vi "Command Engine.vi"(10 "Parameters":variant, 11 "Process":refnum<class "Process.lvclass">) -> ()   [LabVIEW 2015, in "J1939 Addon Engine.lvlib"]
uses:
  J1939 Addon Engine.lvlib
  <vilib>/NI/NIVS Inline Async API/_VS Inline Async API/Process/Process.lvclass
  Types/Diagnostic Data Lookup Table Action.ctl
  <vilib>/NI/NIVS Inline Async API/_VS Inline Async API/Process/Process.lvclass/Process.ctl
  Shared/Types/SysDef Command Settings.ctl
  <vilib>/NI/NIVS Inline Async API/_Data Access Engine/Access Type Classes/Read/Read.lvclass/Read.ctl
  <vilib>/NI/NIVS Inline Async API/_Data Access Engine/Access Type Classes/Write/Write.lvclass/Write.ctl
  APIs/Host Automation API/Types/DTC_Action.ctl
  <vilib>/NI/NIVS Inline Async API/_Data Access Engine/Data Access Engine/Methods/Write.Data.vi
  <vilib>/NI/NIVS Inline Async API/_Data Access Engine/Data Access Engine/Methods/Read.Data.vi
  <vilib>/NI/NIVS Inline Async API/_VS Inline Async API/Process/Data Member Access/Read Data Access.vi
  <vilib>/NI/NIVS Inline Async API/_VS Inline Async API/Error Handling Process/SubVIs/Error.ConvertArray.vi
  <vilib>/NI/NIVS Inline Async API/_Data Access Engine/Access Type Classes/Write/Write.ProcessData.vi
  <vilib>/NI/NIVS Inline Async API/_Data Access Engine/Access Type Classes/Read/Read.ProcessData.vi
  Diagnostic Data Lookup Table.vi
  Shared/SubVIs/Constants.vi
  <vilib>/NI/NIVS Inline Async API/_Data Access Engine/Data Access Engine/Methods/Read.Lookup.vi
  <vilib>/NI/NIVS Inline Async API/_Data Access Engine/Data Access Engine/Methods/Write.Lookup.vi
  <vilib>/NI/NIVS Inline Async API/_Data Access Engine/Data Access Engine/Data Access Engine.lvclass
  APIs/Host Automation API/J1939 Host Automation API.lvlib
  Shared/J1939 Addon Shared.lvlib
  <vilib>/NI Veristand/Custom Device Tools/Custom Device Utility Library/Custom Device Utility Library.lvlib
panel:
  in  "Error":errorcluster
  out "error out":errorcluster
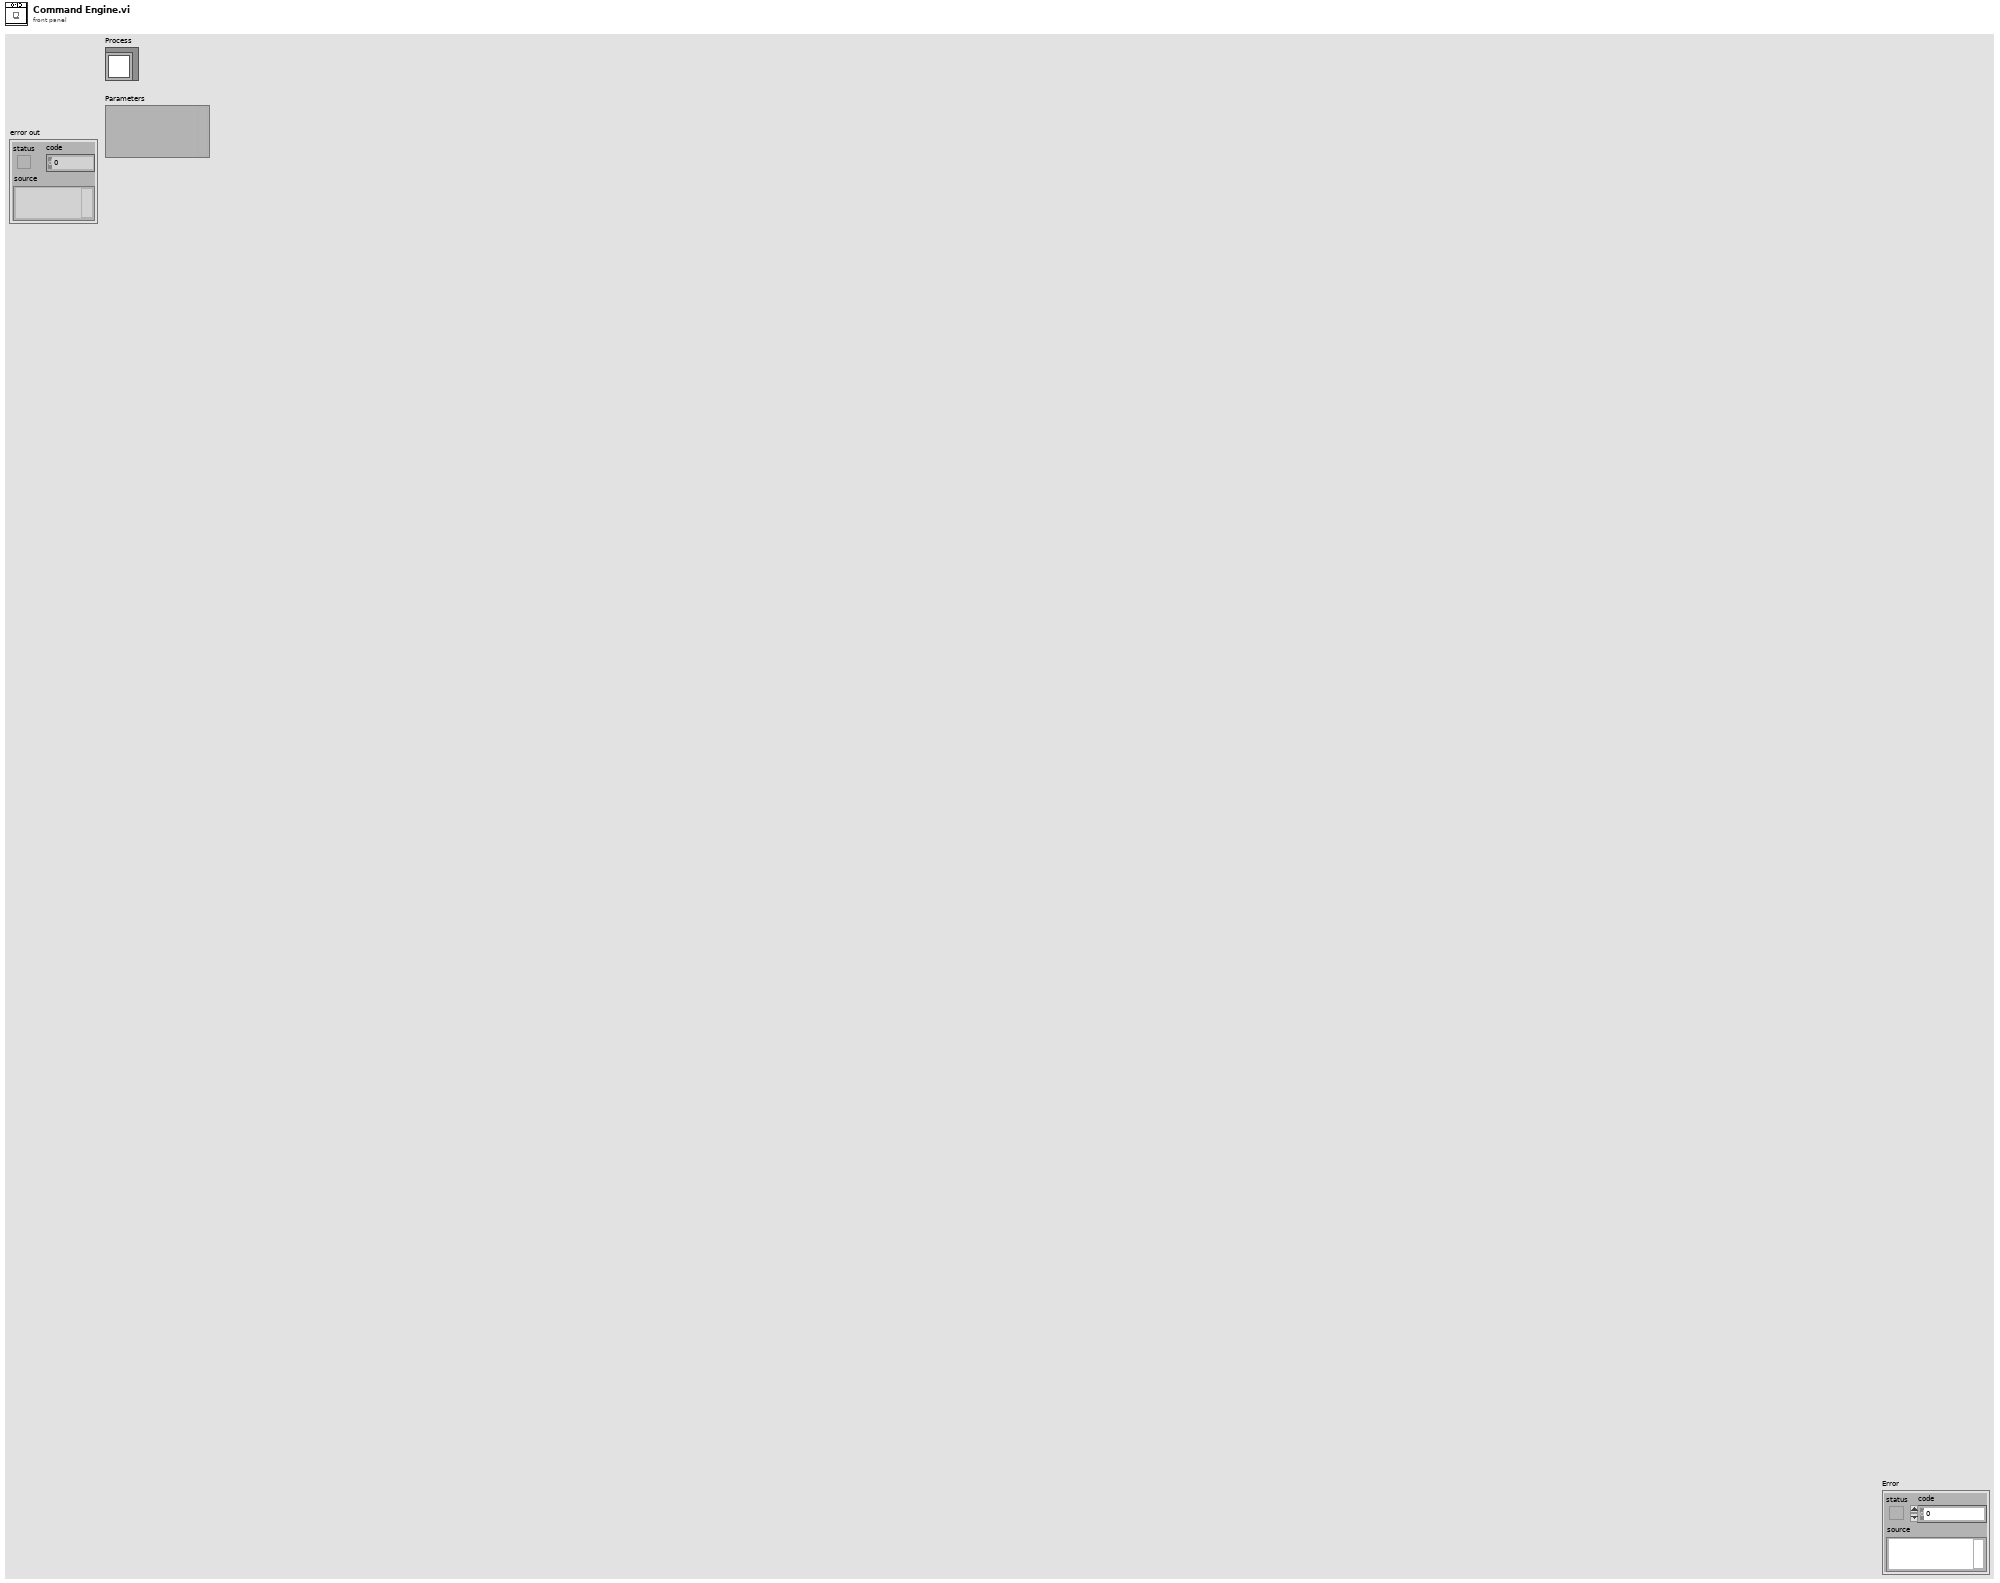
[diagram p1: front panel]
types:
  T1 = typedef "J1939 Addon Shared.lvlib/SysDef Command Settings.ctl" = cluster{"Name":string, "Response Refs":cluster{"Values Array":dbl[], "Response Names":string[]}, "Command Refs":cluster{"Values Array":dbl[], "Command Names":string[]}}
  T2 = typedef "Data Access Engine.lvlib/Data Access Engine.lvclass/Write.DVR.ctl" = refnum<data-value>
  T3 = typedef "Data Access Engine.lvlib/Data Access Engine.lvclass/Read.DVR.ctl" = refnum<data-value>
  T4 = typedef "J1939 Addon Engine.lvlib/Diagnostic Data Lookup Table Reference.ctl" = refnum<data-value>
  T5 = typedef "NI STM.lvlib/TCP Connection Info.ctl" = cluster{"connection ID":refnum<k5>, "meta data":T6[]}
  T6 = typedef "NI STM.lvlib/MetaDataElement.ctl" = string
  T7 = typedef "J1939 Addon Engine.lvlib/Diagnostic Data Lookup Table Action.ctl" = enum16{"Initialize", "Get All", "Set All", "Set Value", "Get Value"}
  T8 = typedef "J1939 Host Automation API.lvlib/DTC_Action.ctl" = enum16{"ALL", "ACTIVE", "INACTIVE"}
  T9 = typedef "J1939 Addon Engine.lvlib/Internal Command Engine States.ctl" = enum8{"Idle", "Refresh Address", "Verify DTCs", "Clear DTCs", "Clear Status Bit", "Clear Error Bit"}
  T10 = typedef "J1939 Host Automation API.lvlib/Verify DTC_Status.ctl" = enum16{"NOT_PRESENT", "ACTIVE", "INACTIVE"}
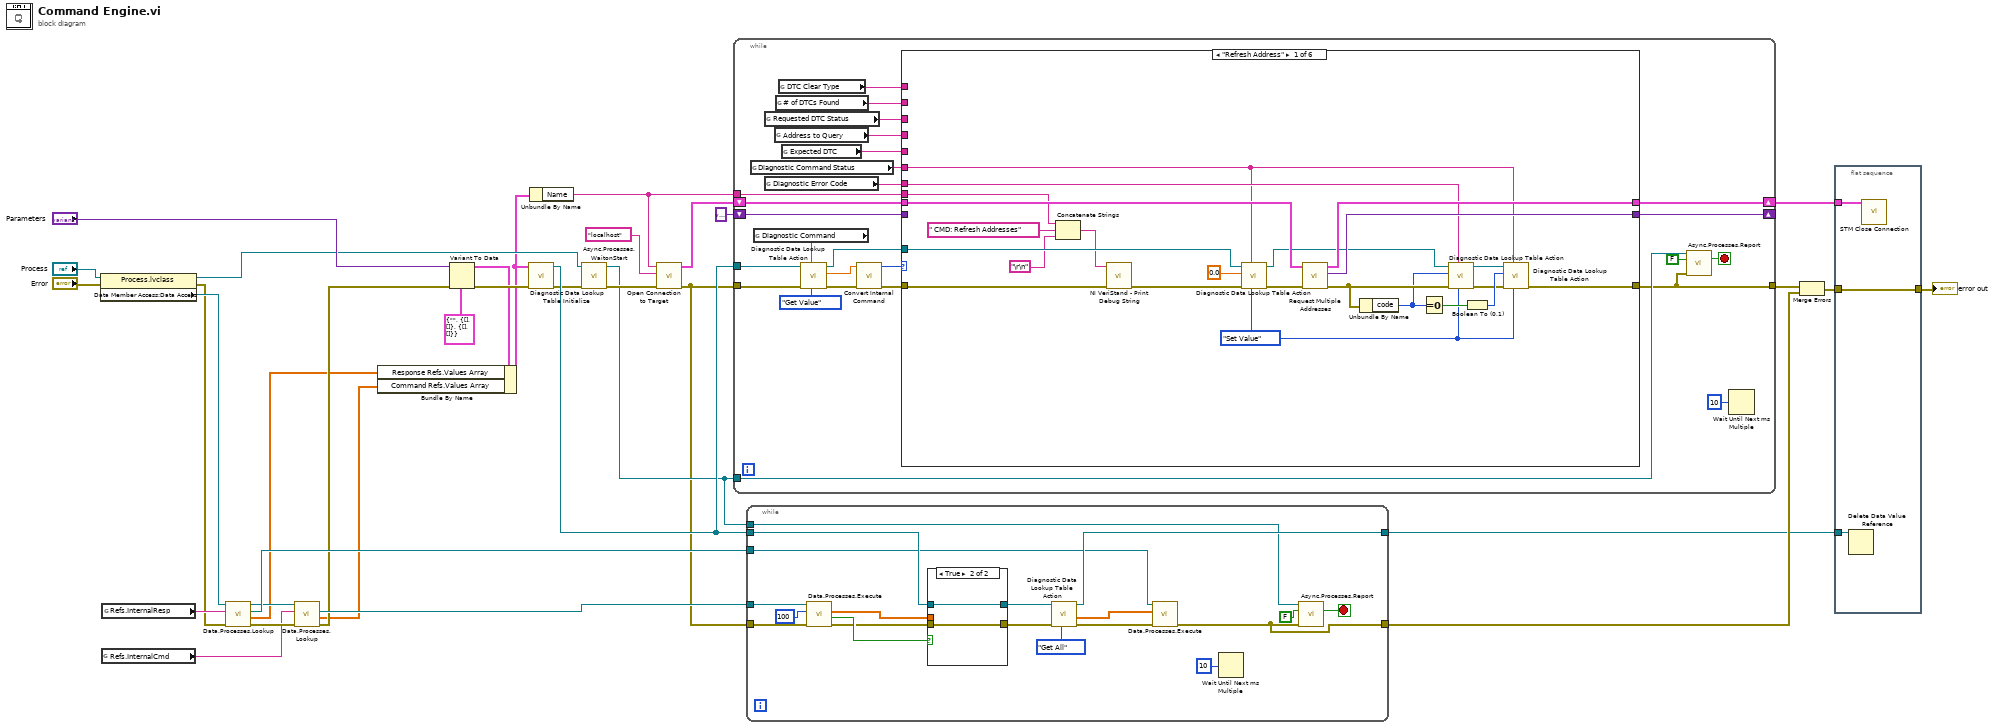
[diagram p0: block diagram]
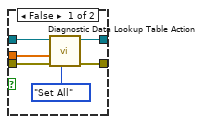
[diagram p2: hidden frame]
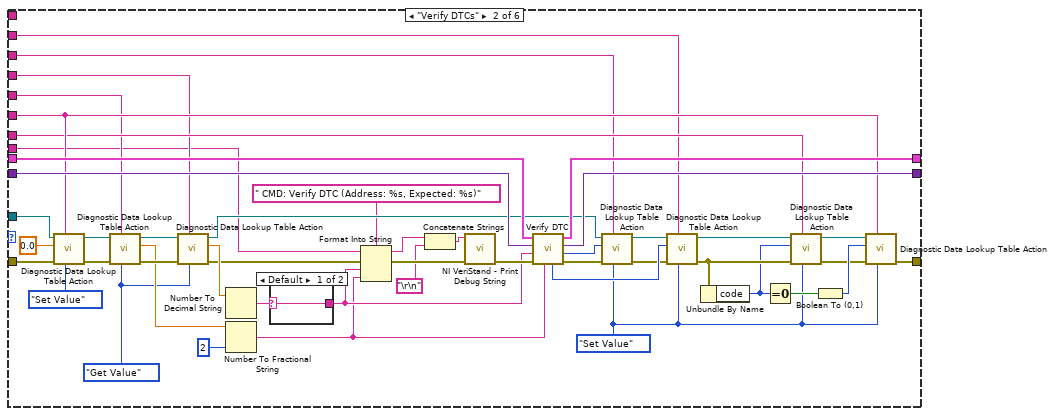
[diagram p3: hidden frame]
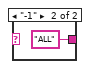
[diagram p4: hidden frame]
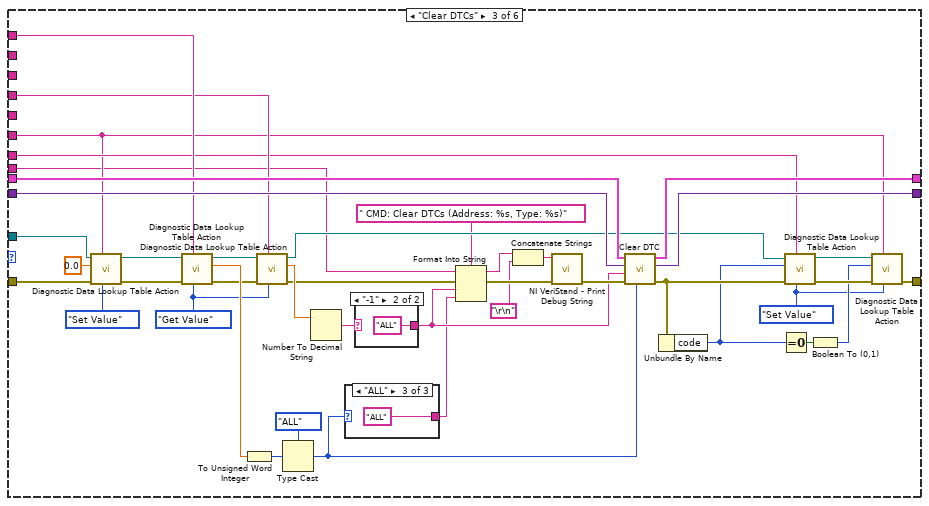
[diagram p5: hidden frame]
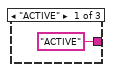
[diagram p6: hidden frame]
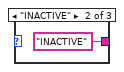
[diagram p7: hidden frame]
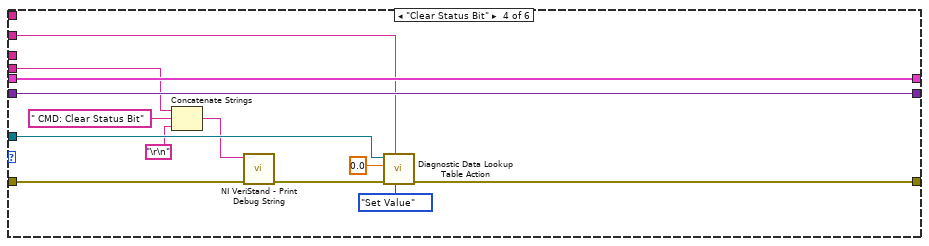
[diagram p9: hidden frame]
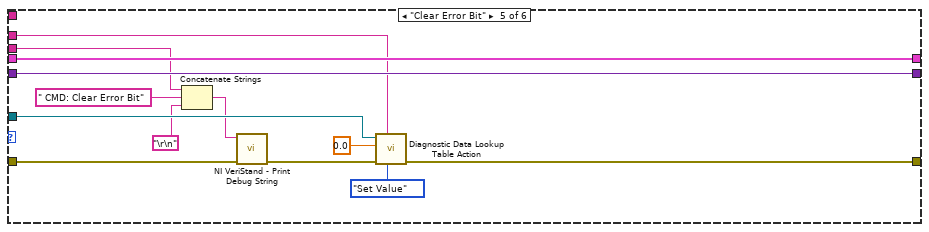
[diagram p10: hidden frame]
diagram:
  n1 = property class="Process.lvclass"(reference="Process", error in="Error") -> (reference out=w18:refnum<class "Process.lvclass">, error out=w10:errorcluster, "Data Member Access:Data Access"=w15:refnum<class "Data Access Engine.lvclass">)
  n2 = global read "Constants.vi" "Refs.InternalCmd"() -> (w13:string)
  n3 = global read "Constants.vi" "Refs.InternalResp"() -> (w12:string)
  n4 = call-poly <vilib>:"Data.Processes.Lookup.vi"("error in (no error)"=w10, "Name"=w12, "Data Access API in"=w15) -> ("error out"=w17:errorcluster, "Initial Values"=w4:dbl[], "Ref"=w20:T2, "Data Access API out"=w16:refnum<class "Data Access Engine.lvclass">)  [unwired: 5 in]
  n5 = call-poly <vilib>:"Data.Processes.Lookup.vi"("error in (no error)"=w17, "Name"=w13, "Data Access API in"=w16) -> ("error out"=w7:errorcluster, "Initial Values"=w3:dbl[], "Ref"=w21:T3)  [unwired: 5 in, 1 out]
  n6 = Variant To Data(error in=w7, type=T1 {"Name"="", "Response Refs"={"Values Array"=[], "Response Names"=[]}, "Command Refs"={"Values Array"=[], "Command Names"=[]}} ("Internal Command Engine References"), Variant="Parameters") -> (data=w5:T1, error out=w8:errorcluster)
  n7 = Bundle By Name(cluster=w5, "Response Refs.Values Array"=w4, "Command Refs.Values Array"=w3) -> (w2:T1)
  n8 = call "Diagnostic Data Lookup Table Initialize.vi"("error in (no error)"=w8, "Internal Command Engine References"=w2) -> ("error out"=w9:errorcluster, "Diag Data Ref"=w31:T4)  [unwired: 8 in]
  n9 = Unbundle By Name(w2) -> ("Name"=w1:string)
  n10 = call <vilib>:"Async.Processes.WaitonStart.vi"("error in (no error)"=w9, "Process"=w18) -> ("error out"=w24:errorcluster, "Process out"=w23:refnum<class "Process.lvclass">)  [unwired: 7 in, 1 out]
  n11 = call "Open Connection to Target.vi"("error in (no error)"=w24, "IP Address"="localhost", "TCP Service"=w1) -> ("error out"=w14:errorcluster, "connection info"=w33:T5)  [unwired: 7 in]
  n12 = while {
    shift-right: [w59] -> _
    shift-left: variant ("Address Lookup Table Out") -> [w58]
    shift-right: [w57] -> w25
    shift-left: w33 -> [w60]
    tunnel: [w35] -> w30
    tunnel: w14 -> [w54]
    tunnel: w23 -> [w52]
    tunnel: w31 -> [w53]
    tunnel: w1 -> [w51]
    stop <- w55 stop-if-true
    n13 = global read "Constants.vi" "Diagnostic Command Status"() -> (w43:string)
    n14 = global read "Constants.vi" "Diagnostic Command"() -> (w45:string)
    n15 = global read "Constants.vi" "Requested DTC Status"() -> (w37:string)
    n16 = global read "Constants.vi" "Diagnostic Error Code"() -> (w41:string)
    n17 = global read "Constants.vi" "Address to Query"() -> (w38:string)
    n18 = global read "Constants.vi" "# of DTCs Found"() -> (w36:string)
    n19 = global read "Constants.vi" "DTC Clear Type"() -> (w40:string)
    n20 = global read "Constants.vi" "Expected DTC"() -> (w39:string)
    n21 = call "Diagnostic Data Lookup Table Action.vi"("command"=Diagnostic_Data_Lookup_Table_Action."Get Value", "Name"=w45, "error in (no error)"=w54, "Diag Data Ref"=w53) -> ("error out"=w47:errorcluster, "Signal Out"=w48:dbl, "Diag Data Ref Out"=w42:T4)  [unwired: 4 in, 1 out]
    n22 = call "Convert Internal Command.vi"("error in (no error)"=w47, "Value"=w48) -> ("error out"=w46:errorcluster, "Enum"=w49:T9)  [unwired: 8 in]
    n23 = case shown="\"Refresh Address\"" w49 {
      tunnel: w60 -> [w83 w131 w175 w192 w205 w208]
      tunnel: [w82 w129 w173 w191 w204 w207] -> w59
      tunnel: w58 -> [_ w130 w174 w191 w204 w207]
      tunnel: [w81 w128 w172 w192 w205 w208] -> w57
      tunnel: w46 -> [w66 w116 w161 w186 w199 w209]
      tunnel: [w76 w112 w163 w190 w203 w209] -> w35
      tunnel: w43 -> [w69 w103 w149 w189 _ _]
      tunnel: w42 -> [w73 w110 w157 w187 w201 _]
      tunnel: w41 -> [w70 w102 w150 _ w202 _]
      tunnel: w40 -> [_ _ w152 _ _ _]
      tunnel: w39 -> [_ w101 _ _ _ _]
      tunnel: w38 -> [_ w100 w151 _ _ _]
      tunnel: w37 -> [_ w99 _ _ _ _]
      tunnel: w36 -> [_ w98 _ _ _ _]
      tunnel: w51 -> [w63 w86 w137 w184 w197 _]
      frame "Refresh Address" {
        w68 = Diagnostic_Data_Lookup_Table_Action."Set Value" ("command")
        n24 = Concatenate Strings(w63, " CMD: Refresh Addresses" ("string"), "\r\n") -> (w62:string)
        n25 = call <vilib>:"NI VeriStand - Print Debug String.vi"("error in (no error)"=w66, "Message"=w62) -> ("error out"=w65:errorcluster)  [unwired: 9 in]
        n26 = call "Diagnostic Data Lookup Table Action.vi"("command"=w68, "Name"=w69, "error in (no error)"=w65, "Signal In"=0.0 ("Value"), "Diag Data Ref"=w73) -> ("error out"=w75:errorcluster, "Diag Data Ref Out"=w72:T4)  [unwired: 3 in, 2 out]
        n27 = call "Request Multiple Addresses.vi"("error in (no error)"=w75, "connection info"=w83) -> ("error out"=w78:errorcluster, "variant"=w82:variant, "connection info"=w81:T5)  [unwired: 6 in, 1 out]
        n28 = Unbundle By Name(w78) -> ("code"=w67:i32)
        n29 = Equal To 0?(x=w67) -> (x = 0?=w80:bool)
        n30 = call "Diagnostic Data Lookup Table Action.vi"("command"=w68, "Name"=w70, "error in (no error)"=w78, "Signal In"=w67, "Diag Data Ref"=w72) -> ("error out"=w77:errorcluster, "Diag Data Ref Out"=w71:T4)  [unwired: 3 in, 2 out]
        n31 = Boolean To (0,1)(Boolean=w80) -> (0, 1=w79:i16)
        n32 = call "Diagnostic Data Lookup Table Action.vi"("command"=w68, "Name"=w69, "error in (no error)"=w77, "Signal In"=w79, "Diag Data Ref"=w71) -> ("error out"=w76:errorcluster)  [unwired: 3 in, 3 out]
      }
      frame "Verify DTCs" {
        w95 = Diagnostic_Data_Lookup_Table_Action."Set Value" ("command")
        w97 = Diagnostic_Data_Lookup_Table_Action."Get Value" ("command")
        n33 = call "Diagnostic Data Lookup Table Action.vi"("command"=Diagnostic_Data_Lookup_Table_Action."Set Value", "Name"=w103, "error in (no error)"=w116, "Signal In"=0.0 ("Value"), "Diag Data Ref"=w110) -> ("error out"=w117:errorcluster, "Diag Data Ref Out"=w109:T4)  [unwired: 3 in, 2 out]
        n34 = call "Diagnostic Data Lookup Table Action.vi"("command"=w97, "Name"=w101, "error in (no error)"=w117, "Diag Data Ref"=w109) -> ("error out"=w125:errorcluster, "Signal Out"=w123:dbl, "Diag Data Ref Out"=w108:T4)  [unwired: 4 in, 1 out]
        n35 = call "Diagnostic Data Lookup Table Action.vi"("command"=w97, "Name"=w100, "error in (no error)"=w125, "Diag Data Ref"=w108) -> ("error out"=w90:errorcluster, "Signal Out"=w127:dbl, "Diag Data Ref Out"=w107:T4)  [unwired: 4 in, 1 out]
        n36 = Number To Decimal String(number=w127) -> (decimal integer string=w126:string)  [unwired: 1 in]
        n37 = Number To Fractional String(number=w123, precision (6)=i16 2) -> (F-format string=w87:string)  [unwired: 2 in]
        n38 = case shown="Default" w126 {
          selector: w126 -> [w132 _]
          tunnel: [w132 "ALL"] -> w88
          frame Default {
          }
          frame "-1" {
          }
        }
        n39 = Format Into String(format string=" CMD: Verify DTC (Address: %s, Expected: %s)" ("string"), initial string=w86, error in=w90, w88, w87) -> (resulting string=w92:string, error out=w91:errorcluster)
        n40 = Concatenate Strings(w92, "\r\n") -> (w85:string)
        n41 = call <vilib>:"NI VeriStand - Print Debug String.vi"("error in (no error)"=w91, "Message"=w85) -> ("error out"=w89:errorcluster)  [unwired: 9 in]
        n42 = call "Verify DTC.vi"("Expected DTC"=w87, "error in"=w89, "Address"=w88, "Address Lookup Table"=w130, "connection info"=w131) -> ("error out"=w114:errorcluster, "Status"=w121:T10, "Address Lookup Table Out"=w129:variant, "connection info"=w128:T5, "Found DTCs"=w122:i32)  [unwired: 2 in]
        n43 = call "Diagnostic Data Lookup Table Action.vi"("command"=w95, "Name"=w99, "error in (no error)"=w114, "Signal In"=w121, "Diag Data Ref"=w107) -> ("error out"=w115:errorcluster, "Diag Data Ref Out"=w106:T4)  [unwired: 3 in, 2 out]
        n44 = call "Diagnostic Data Lookup Table Action.vi"("command"=w95, "Name"=w98, "error in (no error)"=w115, "Signal In"=w122, "Diag Data Ref"=w106) -> ("error out"=w111:errorcluster, "Diag Data Ref Out"=w105:T4)  [unwired: 3 in, 2 out]
        n45 = Unbundle By Name(w111) -> ("code"=w94:i32)
        n46 = Equal To 0?(x=w94) -> (x = 0?=w120:bool)
        n47 = call "Diagnostic Data Lookup Table Action.vi"("command"=w95, "Name"=w102, "error in (no error)"=w111, "Signal In"=w94, "Diag Data Ref"=w105) -> ("error out"=w113:errorcluster, "Diag Data Ref Out"=w104:T4)  [unwired: 3 in, 2 out]
        n48 = Boolean To (0,1)(Boolean=w120) -> (0, 1=w119:i16)
        n49 = call "Diagnostic Data Lookup Table Action.vi"("command"=w95, "Name"=w103, "error in (no error)"=w113, "Signal In"=w119, "Diag Data Ref"=w104) -> ("error out"=w112:errorcluster)  [unwired: 3 in, 3 out]
      }
      frame "Clear DTCs" {
        w146 = Diagnostic_Data_Lookup_Table_Action."Set Value" ("command")
        w147 = Diagnostic_Data_Lookup_Table_Action."Get Value" ("command")
        n50 = call "Diagnostic Data Lookup Table Action.vi"("command"=Diagnostic_Data_Lookup_Table_Action."Set Value", "Name"=w149, "error in (no error)"=w161, "Signal In"=0.0 ("Value"), "Diag Data Ref"=w157) -> ("error out"=w159:errorcluster, "Diag Data Ref Out"=w156:T4)  [unwired: 3 in, 2 out]
        n51 = call "Diagnostic Data Lookup Table Action.vi"("command"=w147, "Name"=w152, "error in (no error)"=w159, "Diag Data Ref"=w156) -> ("error out"=w158:errorcluster, "Signal Out"=w169:dbl, "Diag Data Ref Out"=w155:T4)  [unwired: 4 in, 1 out]
        n52 = To Unsigned Word Integer(number=w169) -> (unsigned 16bit integer=w168:u16)
        n53 = call "Diagnostic Data Lookup Table Action.vi"("command"=w147, "Name"=w151, "error in (no error)"=w158, "Diag Data Ref"=w155) -> ("error out"=w141:errorcluster, "Signal Out"=w171:dbl, "Diag Data Ref Out"=w154:T4)  [unwired: 4 in, 1 out]
        n54 = Type Cast(type=DTC_Action."ALL" ("Action"), x=w168) -> (*(type *) &x=w143:T8)
        n55 = Number To Decimal String(number=w171) -> (decimal integer string=w170:string)  [unwired: 1 in]
        n56 = case shown="\"ALL\"" w143 {
          tunnel: ["ACTIVE" "INACTIVE" "ALL"] -> w138
          frame "ACTIVE" {
          }
          frame "INACTIVE" {
          }
          frame "ALL" {
          }
        }
        n57 = case shown="\"-1\"" w170 {
          selector: w170 -> [w179 _]
          tunnel: [w179 "ALL"] -> w139
          frame Default {
          }
          frame "-1" {
          }
        }
        n58 = Format Into String(format string=" CMD: Clear DTCs (Address: %s, Type: %s)" ("string"), initial string=w137, error in=w141, w139, w138) -> (resulting string=w135:string, error out=w142:errorcluster)
        n59 = Concatenate Strings(w135, "\r\n") -> (w134:string)
        n60 = call <vilib>:"NI VeriStand - Print Debug String.vi"("error in (no error)"=w142, "Message"=w134) -> ("error out"=w140:errorcluster)  [unwired: 9 in]
        n61 = call "Clear DTC.vi"("Action"=w143, "error in"=w140, "Address (ALL)"=w139, "Address Lookup Table"=w174, "connection info"=w175) -> ("error out"=w164:errorcluster, "Address Lookup Table Out"=w173:variant, "connection info"=w172:T5)  [unwired: 4 in]
        n62 = Unbundle By Name(w164) -> ("code"=w145:i32)
        n63 = Equal To 0?(x=w145) -> (x = 0?=w166:bool)
        n64 = call "Diagnostic Data Lookup Table Action.vi"("command"=w146, "Name"=w150, "error in (no error)"=w164, "Signal In"=w145, "Diag Data Ref"=w154) -> ("error out"=w165:errorcluster, "Diag Data Ref Out"=w153:T4)  [unwired: 3 in, 2 out]
        n65 = Boolean To (0,1)(Boolean=w166) -> (0, 1=w160:i16)
        n66 = call "Diagnostic Data Lookup Table Action.vi"("command"=w146, "Name"=w149, "error in (no error)"=w165, "Signal In"=w160, "Diag Data Ref"=w153) -> ("error out"=w163:errorcluster)  [unwired: 3 in, 3 out]
      }
      frame "Clear Status Bit" {
        n67 = Concatenate Strings(w184, " CMD: Clear Status Bit" ("string"), "\r\n") -> (w182:string)
        n68 = call <vilib>:"NI VeriStand - Print Debug String.vi"("error in (no error)"=w186, "Message"=w182) -> ("error out"=w185:errorcluster)  [unwired: 9 in]
        n69 = call "Diagnostic Data Lookup Table Action.vi"("command"=Diagnostic_Data_Lookup_Table_Action."Set Value", "Name"=w189, "error in (no error)"=w185, "Signal In"=0.0 ("Value"), "Diag Data Ref"=w187) -> ("error out"=w190:errorcluster)  [unwired: 3 in, 3 out]
      }
      frame "Clear Error Bit" {
        n70 = Concatenate Strings(w197, " CMD: Clear Error Bit" ("string"), "\r\n") -> (w195:string)
        n71 = call <vilib>:"NI VeriStand - Print Debug String.vi"("error in (no error)"=w199, "Message"=w195) -> ("error out"=w198:errorcluster)  [unwired: 9 in]
        n72 = call "Diagnostic Data Lookup Table Action.vi"("command"=Diagnostic_Data_Lookup_Table_Action."Set Value", "Name"=w202, "error in (no error)"=w198, "Signal In"=0.0 ("Value"), "Diag Data Ref"=w201) -> ("error out"=w203:errorcluster)  [unwired: 3 in, 3 out]
      }
      frame "Idle" {
      }
    }
    n73 = call <vilib>:"Async.Processes.Report.vi"("Error"=w35, "Stop Async on Error?"=FALSE ("Stop on Error?"), "Process in"=w52) -> ("Stop"=w55:bool)  [unwired: 7 in, 1 out]
    n74 = Wait Until Next ms Multiple(millisecond multiple=u32 10) -> ()  [unwired: 1 out]
  }
  n75 = while {
    tunnel: w31 -> [w226]
    tunnel: [w212] -> w29
    tunnel: w23 -> [w224]
    tunnel: w14 -> [w215]
    tunnel: [w225] -> w26
    tunnel: w21 -> [w216]
    tunnel: w20 -> [w214]
    stop <- w227 stop-if-true
    n76 = call-poly <vilib>:"Data.Processes.Execute.vi"("error in (no error)"=w215, "timeout ms"=100 ("timeout in ms (0)"), "Ref"=w216) -> ("error out"=w210:errorcluster, "Timeout?"=w217:bool, "Values"=w218:dbl[])  [unwired: 6 in]
    n77 = case shown="True" w217 {
      tunnel: w218 -> [w229 _]
      tunnel: w210 -> [w233 w236]
      tunnel: [w232 w236] -> w221
      tunnel: w226 -> [w231 w235]
      tunnel: [w230 w235] -> w220
      frame False {
        n78 = call "Diagnostic Data Lookup Table Action.vi"("command"=Diagnostic_Data_Lookup_Table_Action."Set All", "error in (no error)"=w233, "Signals"=w229, "Diag Data Ref"=w231) -> ("error out"=w232:errorcluster, "Diag Data Ref Out"=w230:T4)  [unwired: 4 in, 2 out]
      }
      frame True {
      }
    }
    n79 = call "Diagnostic Data Lookup Table Action.vi"("command"=Diagnostic_Data_Lookup_Table_Action."Get All", "error in (no error)"=w221, "Diag Data Ref"=w220) -> ("error out"=w211:errorcluster, "Signals Out"=w213:dbl[], "Diag Data Ref Out"=w225:T4)  [unwired: 5 in, 1 out]
    n80 = call-poly <vilib>:"Data.Processes.Execute.vi"("error in (no error)"=w211, "Values"=w213, "Ref"=w214) -> ("error out"=w212:errorcluster)  [unwired: 8 in]
    n81 = Wait Until Next ms Multiple(millisecond multiple=u32 10) -> ()  [unwired: 1 out]
    n82 = call <vilib>:"Async.Processes.Report.vi"("Error"=w212, "Stop Async on Error?"=FALSE ("Stop on Error?"), "Process in"=w224) -> ("Stop"=w227:bool)  [unwired: 7 in, 1 out]
  }
  n83 = Merge Errors(w30, w29) -> (w27:errorcluster)
  n84 = flat-sequence {
    tunnel: [w239] -> w28
    tunnel: w27 -> [w239]
    tunnel: w26 -> [w238]
    tunnel: w25 -> [w237]
    frame #0 {
      n85 = Delete Data Value Reference(data value reference=w238) -> ()  [unwired: 1 in, 2 out]
      n86 = call "STM Close Connection.vi"("connection info"=w237) -> ()  [unwired: 10 in, 1 out]
    }
  }
  "error out" <- w28
